vi "Close.vi"(0 "comm interface in":refnum<class "RoboRIO SPI.lvclass">, 11 "error in":errorcluster) -> (15 "error out":errorcluster)   [LabVIEW 2018, in "RoboRIO SPI.lvclass"]
uses:
  RoboRIO SPI.lvclass
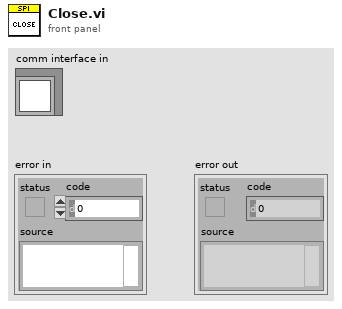
[diagram p1: front panel]
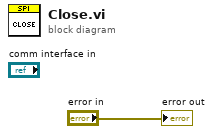
[diagram p0: block diagram]
diagram:
  "error out" <- "error in"
